vi "Comandos de movimiento micrometrico Z.vi"(3 "error in":errorcluster, 4 "VISA in":refnum<visa-resource-name>, 5 "Micras en Z":dbl, 6 "Activar Movimiento en Z":bool) -> (0 "error out":errorcluster, 1 "VISA out":refnum<visa-resource-name>, 2 "Siguiente caso":i32)   [LabVIEW 2018]
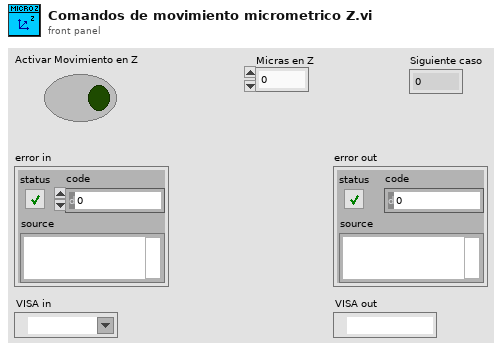
[diagram p1: front panel]
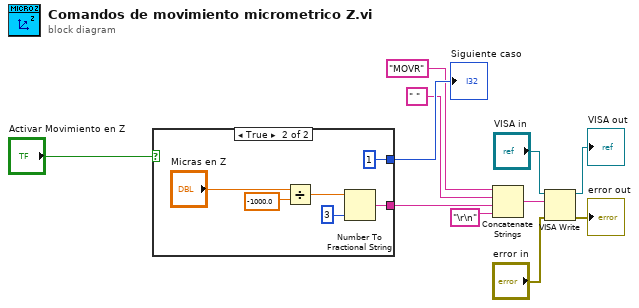
[diagram p0: block diagram]
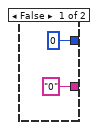
[diagram p2: hidden frame]
diagram:
  n1 = case shown="True" "Activar Movimiento en Z" {
    tunnel: ["0" w16] -> w3
    tunnel: [0 1] -> w10
    frame False {
    }
    frame True {
      n2 = Divide(x="Micras en Z", y=-1000.0) -> (x/y=w17:dbl)
      n3 = Number To Fractional String(number=w17, precision (6)=i16 3) -> (F-format string=w16:string)  [unwired: 2 in]
    }
  }
  "Siguiente caso" <- w10
  n4 = Concatenate Strings("MOVR" ("string"), " " ("string"), w3, "\r\n" ("string")) -> (w2:string)
  n5 = VISA Write(VISA resource name="VISA in", write buffer=w2, error in (no error)="error in") -> (VISA resource name out=→"VISA out":refnum<visa-resource-name>, error out=→"error out":errorcluster)  [unwired: 1 out]
